vi "HISTOGRAMA.vi"(1 "Array":u8[][](array[numeric])) -> (0 "Waveform Graph":dbl[](graph))   [LabVIEW 2020]
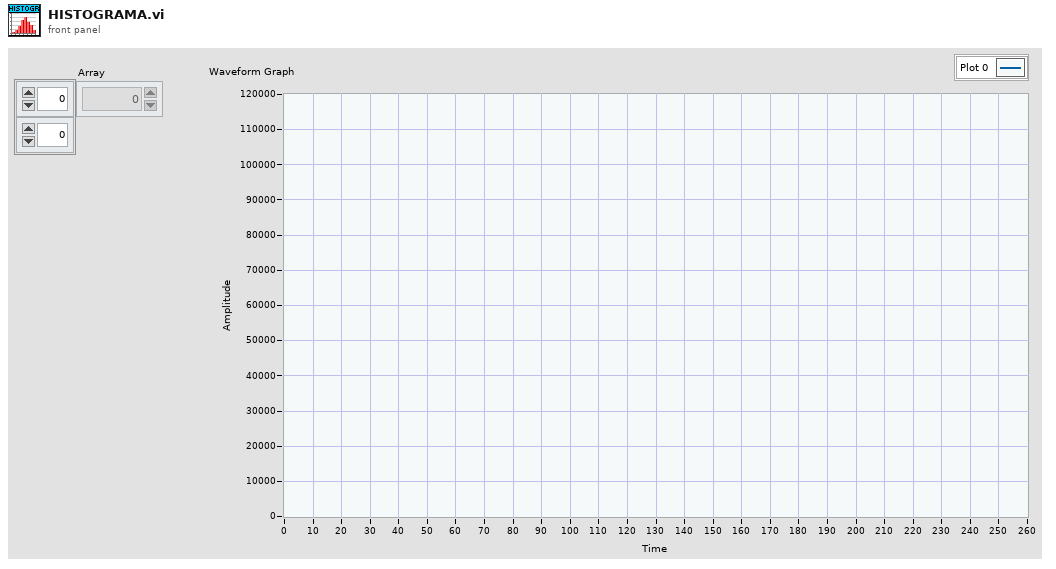
[diagram p1: front panel]
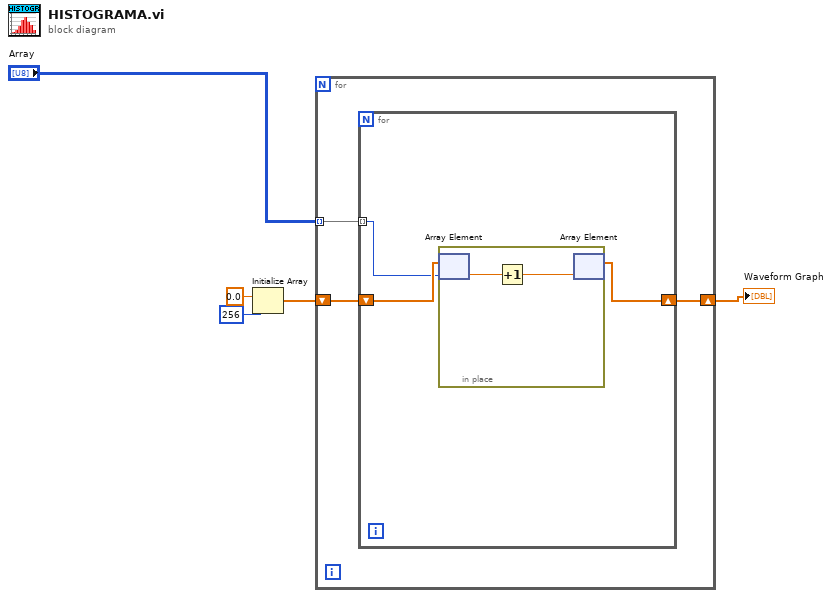
[diagram p0: block diagram]
diagram:
  n1 = Initialize Array(0.0 ("element"), 256 ("dimension size")) -> (w4:dbl[])
  n2 = for {
    tunnel: "Array" -> [w8] mode=indexing
    shift-right: [w6] -> w5
    shift-left: w4 -> [w7]
    n3 = for {
      tunnel: w8 -> [w10] mode=indexing
      shift-right: [w9] -> w6
      shift-left: w7 -> [w11]
      n4 = in-place {
        n5 = in-place-array #1(w11, w10) -> (w13:dbl)
        n6 = Increment(x=w13) -> (x+1=w12:dbl)
        n7 = in-place-array #1(w12) -> (w9:dbl[])  [unwired: 1 out]
      }
    }
  }
  "Waveform Graph" <- w5
